vi "Read VI Ref.vi"(8 "error in (no error)":errorcluster, 11 "Graph Manager in":refnum<class "Display Abstract.lvclass">) -> (0 "error out":errorcluster, 2 "VI Ref":refnum<vi>, 3 "Graph Manager out":refnum<class "Display Abstract.lvclass">)   [LabVIEW 2021, in "Display Abstract.lvclass"]
doc: "Do nothing."
uses:
  Display Abstract.lvclass
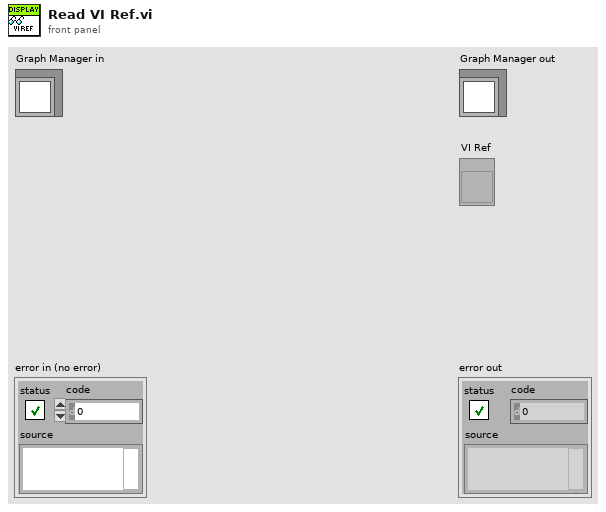
[diagram p1: front panel]
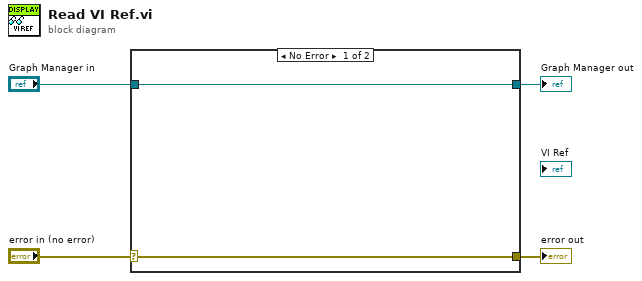
[diagram p0: block diagram]
diagram:
  n1 = case shown="No Error" "error in (no error)" {
    selector: "error in (no error)" -> [w6 w7]
    tunnel: [w6 w7] -> w3
    tunnel: [w5 w8] -> w1
    tunnel: "Graph Manager in" -> [w5 w8]
    frame No Error {
    }
    frame Error {
    }
  }
  "error out" <- w3
  "Graph Manager out" <- w1
